vi "Calculate_Theta.vi"(6 "Center":cluster{"X":dbl, "Y":dbl}, 8 "error in":errorcluster, 10 "Destination":cluster{"X":dbl, "Y":dbl}, 11 "Position":cluster{"X":dbl, "Y":dbl}) -> (0 "error out":errorcluster, 2 "Theta":dbl)   [LabVIEW 2017]
doc: "Calculates the angle between two axes based on a center point."
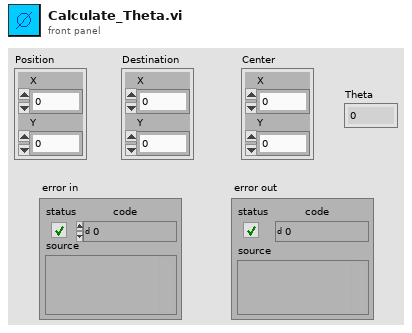
[diagram p1: front panel]
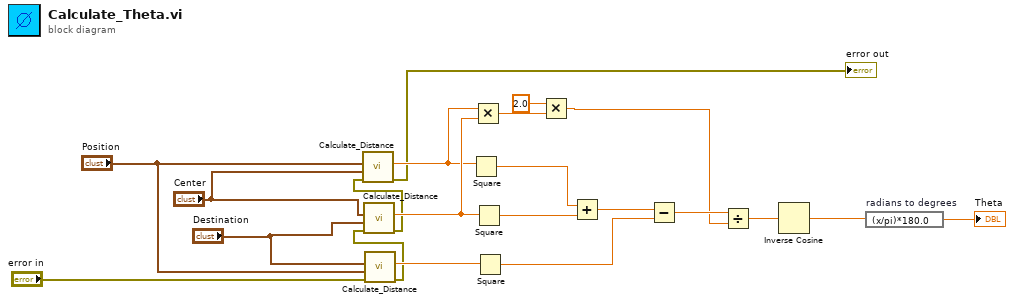
[diagram p0: block diagram]
diagram:
  n1 = call "Calculate_Distance.vi"("error in (no error)"="error in", "B"="Position", "A"="Destination") -> ("error out"=w5:errorcluster, "Distance"=w21:dbl)  [unwired: 7 in]
  n2 = call "Calculate_Distance.vi"("error in (no error)"=w5, "B"="Destination", "A"="Center") -> ("error out"=w4:errorcluster, "Distance"=w17:dbl)  [unwired: 7 in]
  n3 = call "Calculate_Distance.vi"("error in (no error)"=w4, "B"="Center", "A"="Position") -> ("error out"=→"error out":errorcluster, "Distance"=w16:dbl)  [unwired: 7 in]
  n4 = Square(x=w16) -> (x^2=w12:dbl)
  n5 = Multiply(x=w16, y=w17) -> (x*y=w15:dbl)
  n6 = Square(x=w17) -> (x^2=w13:dbl)
  n7 = Square(x=w21) -> (x^2=w10:dbl)
  n8 = Multiply(x=2.0, y=w15) -> (x*y=w8:dbl)
  n9 = Add(x=w12, y=w13) -> (x+y=w11:dbl)
  n10 = Subtract(x=w11, y=w10) -> (x-y=w9:dbl)
  n11 = Divide(x=w9, y=w8) -> (x/y=w7:dbl)
  n12 = Inverse Cosine(1:w7) -> (0:w2:dbl)
  n13 = expression code="(x/pi)*180.0" "radians to degrees"(w2) -> (→"Theta":dbl)
